vi "流程汇总.vi"(11 "参数":T1) -> ()   [LabVIEW 2016, in "质控单元.lvlib"]
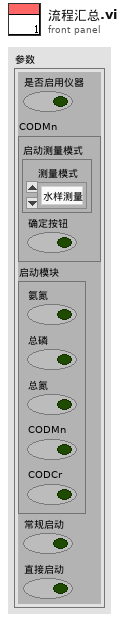
[diagram p1: front panel]
types:
  T1 = cluster{"是否启用仪器":bool, "CODMn":cluster{"启动测量模式":cluster{"测量模式":enum16{"水样测量", "标样核查", "加标回收", "平行样", "校零", "校标"}}, "确定按钮":bool}, "启动模块":cluster{"氨氮":bool, "总磷":bool, "总氮":bool, "CODMn":bool, "CODCr":bool}, "常规启动":bool, "直接启动":bool}
  T2 = enum32{"Bad", "Idle", "Run top level", "Running"}
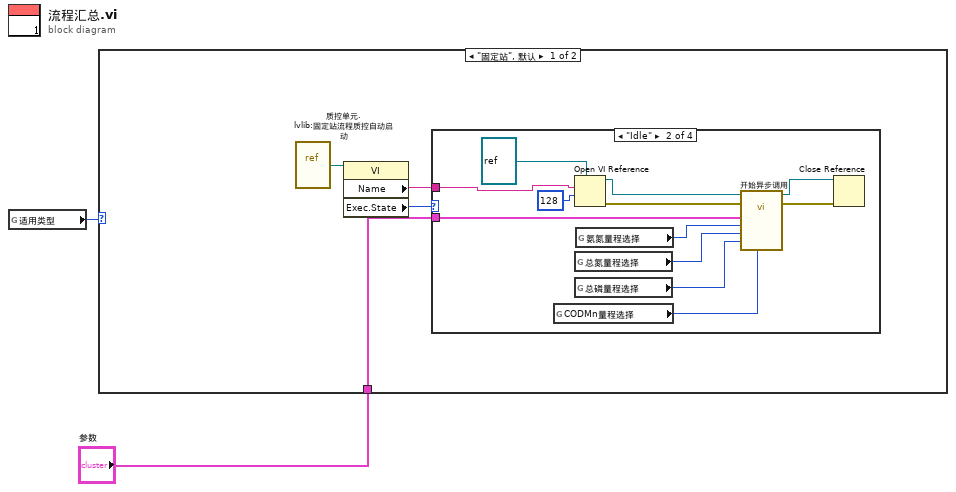
[diagram p0: block diagram]
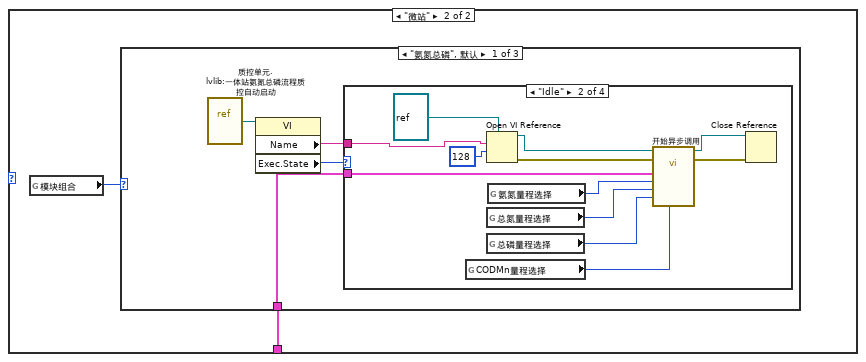
[diagram p5: hidden frame]
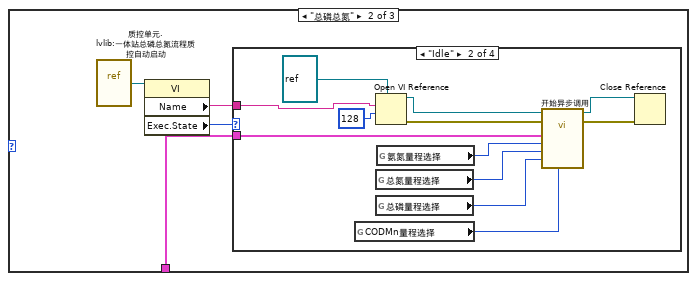
[diagram p9: hidden frame]
diagram:
  n1 = global read "断电保存全局.vi" "适用类型"() -> (w1:enum16{"固定站", "微站"})
  n2 = case shown="\"固定站\", 默认" w1 {
    tunnel: "参数" -> [w3 w19]
    frame "固定站", Default {
      n3 = vi-ref "质控单元.lvlib:固定站流程质控自动启动.vi"() -> (w5:refnum<vi>)
      n4 = property class="VI"(reference=w5) -> ("Name"=w6:string, "Exec.State"=w4:T2)  [unwired: 1 in, 2 out]
      n5 = case shown="\"Idle\"" w4 {
        tunnel: w6 -> [_ w17 _ _]
        tunnel: w3 -> [_ w7 _ _]
        frame "Bad", Default {
        }
        frame "Idle" {
          n6 = global read "断电保存全局.vi" "CODMn量程选择"() -> (w11:enum32{"H", "L", "AUTO"})
          n7 = Open VI Reference(type specifier VI Refnum (for type only)=refnum<vi> refnum ("类型说明符VI引用句柄（仅用于类型）"), vi path=w17, options=128 ("选项")) -> (vi reference=w18:refnum<vi>, error out=w14:errorcluster)  [unwired: 3 in]
          n8 = global read "断电保存全局.vi" "总氮量程选择"() -> (w9:enum32{"H", "L", "AUTO"})
          n9 = global read "断电保存全局.vi" "总磷量程选择"() -> (w10:enum32{"H", "L", "AUTO"})
          n10 = global read "断电保存全局.vi" "氨氮量程选择"() -> (w8:enum32{"H", "L", "AUTO"})
          n11 = call-by-ref "开始异步调用"(reference=w18, error in=w14, "CODMn量程切换"=w11, "总磷量程切换"=w10, "总氮量程切换"=w9, "氨氮量程切换"=w8, "参数"=w7) -> (reference out=w16:refnum<vi>, error out=w15:errorcluster)  [unwired: 7 in]
          n12 = Close Reference(reference=w16, error in (no error)=w15) -> ()  [unwired: 1 out]
        }
        frame "Run top level" {
        }
        frame "Running" {
        }
      }
    }
    frame "微站" {
      n13 = global read "断电保存全局.vi" "模块组合"() -> (w20:enum16{"氨氮总磷", "总磷总氮", "氨氮、总磷、总氮"})
      n14 = case shown="\"氨氮总磷\", 默认" w20 {
        tunnel: w19 -> [w21 w37 _]
        frame "氨氮总磷", Default {
          n15 = vi-ref "质控单元.lvlib:一体站氨氮总磷流程质控自动启动.vi"() -> (w23:refnum<vi>)
          n16 = property class="VI"(reference=w23) -> ("Name"=w24:string, "Exec.State"=w22:T2)  [unwired: 1 in, 2 out]
          n17 = case shown="\"Idle\"" w22 {
            tunnel: w24 -> [_ w35 _ _]
            tunnel: w21 -> [_ w25 _ _]
            frame "Bad", Default {
            }
            frame "Idle" {
              n18 = global read "断电保存全局.vi" "CODMn量程选择"() -> (w29:enum32{"H", "L", "AUTO"})
              n19 = Open VI Reference(type specifier VI Refnum (for type only)=refnum<vi> refnum ("类型说明符VI引用句柄（仅用于类型）"), vi path=w35, options=128 ("选项")) -> (vi reference=w36:refnum<vi>, error out=w32:errorcluster)  [unwired: 3 in]
              n20 = global read "断电保存全局.vi" "总氮量程选择"() -> (w27:enum32{"H", "L", "AUTO"})
              n21 = global read "断电保存全局.vi" "总磷量程选择"() -> (w28:enum32{"H", "L", "AUTO"})
              n22 = global read "断电保存全局.vi" "氨氮量程选择"() -> (w26:enum32{"H", "L", "AUTO"})
              n23 = call-by-ref "开始异步调用"(reference=w36, error in=w32, "CODMn量程切换"=w29, "总磷量程切换"=w28, "总氮量程切换"=w27, "氨氮量程切换"=w26, "参数"=w25) -> (reference out=w34:refnum<vi>, error out=w33:errorcluster)  [unwired: 7 in]
              n24 = Close Reference(reference=w34, error in (no error)=w33) -> ()  [unwired: 1 out]
            }
            frame "Run top level" {
            }
            frame "Running" {
            }
          }
        }
        frame "总磷总氮" {
          n25 = vi-ref "质控单元.lvlib:一体站总磷总氮流程质控自动启动.vi"() -> (w39:refnum<vi>)
          n26 = property class="VI"(reference=w39) -> ("Name"=w40:string, "Exec.State"=w38:T2)  [unwired: 1 in, 2 out]
          n27 = case shown="\"Idle\"" w38 {
            tunnel: w40 -> [_ w51 _ _]
            tunnel: w37 -> [_ w43 _ _]
            frame "Bad", Default {
            }
            frame "Idle" {
              n28 = global read "断电保存全局.vi" "CODMn量程选择"() -> (w41:enum32{"H", "L", "AUTO"})
              n29 = Open VI Reference(type specifier VI Refnum (for type only)=refnum<vi> refnum ("类型说明符VI引用句柄（仅用于类型）"), vi path=w51, options=128 ("选项")) -> (vi reference=w52:refnum<vi>, error out=w48:errorcluster)  [unwired: 3 in]
              n30 = global read "断电保存全局.vi" "总氮量程选择"() -> (w44:enum32{"H", "L", "AUTO"})
              n31 = global read "断电保存全局.vi" "总磷量程选择"() -> (w45:enum32{"H", "L", "AUTO"})
              n32 = global read "断电保存全局.vi" "氨氮量程选择"() -> (w42:enum32{"H", "L", "AUTO"})
              n33 = call-by-ref "开始异步调用"(reference=w52, error in=w48, "CODMn量程切换"=w41, "总磷量程切换"=w45, "总氮量程切换"=w44, "氨氮量程切换"=w42, "参数"=w43) -> (reference out=w50:refnum<vi>, error out=w49:errorcluster)  [unwired: 7 in]
              n34 = Close Reference(reference=w50, error in (no error)=w49) -> ()  [unwired: 1 out]
            }
            frame "Run top level" {
            }
            frame "Running" {
            }
          }
        }
        frame "氨氮、总磷、总氮" {
        }
      }
    }
  }
